vi "big2little.vi"(1 "BigEndian":u32 format="%08x") -> (0 "SmallEndian":u32 format="%08x")   [LabVIEW 2015]
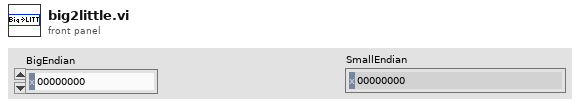
[diagram p1: front panel]
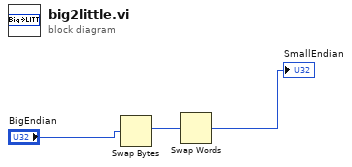
[diagram p0: block diagram]
diagram:
  n1 = Swap Bytes(anything="BigEndian") -> (byte swapped=w2:u32)
  n2 = Swap Words(1:w2) -> (0:→"SmallEndian":u32)
